vi "Text Sections Get Pixel Number.vi"(8 "Error In":errorcluster, 10 "Line Numbers":T1, 11 "Rows where whitespace starts":i32[](array[numeric])) -> (0 "Error Out":errorcluster, 1 "Footer":i32, 2 "Header":i32, 3 "Line Pixel Value (Vertical)":T1, 4 "Main":i32)   [LabVIEW 2018, in "Receipt Parsing.lvlib"]
uses:
  Receipt Parsing.lvlib
  Line Number.ctl
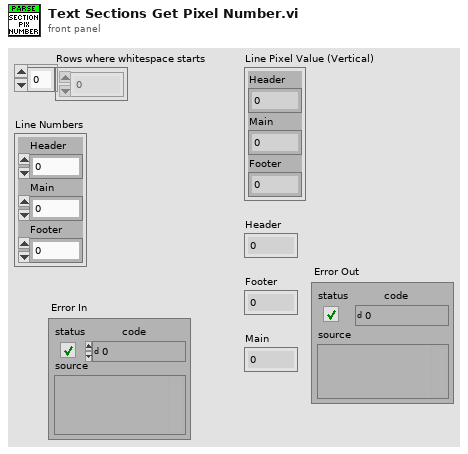
[diagram p1: front panel]
types:
  T1 = typedef "Receipt Parsing.lvlib/Line Number.ctl" = cluster{"Header":i32, "Main":i32, "Footer":i32}
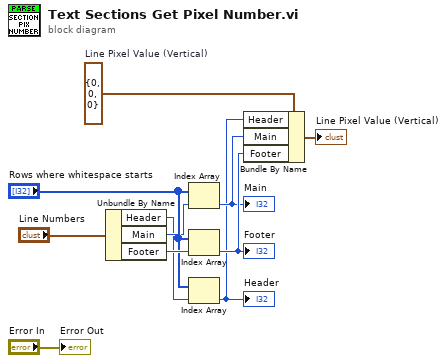
[diagram p0: block diagram]
diagram:
  w7 = T1 {"Header"=0, "Main"=0, "Footer"=0}  # Line Pixel Value (Vertical)
  n1 = Unbundle By Name("Line Numbers") -> ("Header"=w3:i32, "Main"=w4:i32, "Footer"=w6:i32)
  n2 = Index Array(array="Rows where whitespace starts", index=w4) -> (element=w9:i32)
  "Main" <- w9
  n3 = Index Array(array="Rows where whitespace starts", index=w6) -> (element=w10:i32)
  "Footer" <- w10
  n4 = Index Array(array="Rows where whitespace starts", index=w3) -> (element=w8:i32)
  "Header" <- w8
  n5 = Bundle By Name(cluster=w7, "Header"=w8, "Main"=w9, "Footer"=w10) -> (→"Line Pixel Value (Vertical)":T1)
  "Error Out" <- "Error In"
